vi "Measure S-Param.vi"(4 "error in (no error)":errorcluster, 5 "Array":T1[](array[typedef])=[enum."S11", enum."S12", enum."S21", enum."S22"], 6 "DataFile":path, 7 "Data in":T2 {"LogStartTime" format="%<%x %.3X>T"}) -> (0 "error out":errorcluster, 1 "FileSaved":bool, 3 "Data Out out":T2 {"LogStartTime" format="%<%x %.3X>T"})   [LabVIEW 2023]
uses:
  controls/UI Data.ctl
  <vilib>/NI/Modbus Library/API/Master/Modbus Master.lvclass
  LibreVNA/LibreVNA.lvclass
  LibreVNA/Types/Trace Enum.ctl
  <userlib>/_OpenG.lib/time/time.llb/openg_time.lvlib
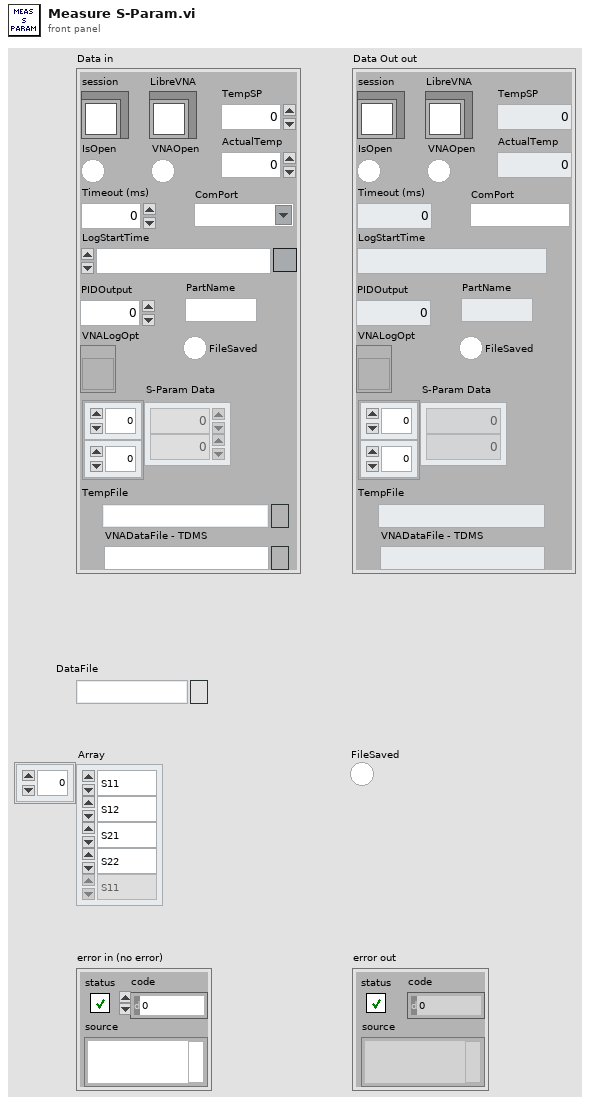
[diagram p1: front panel]
types:
  T1 = typedef "LibreVNA.lvclass/Trace Enum.ctl" = enum16{"S11", "S12", "S21", "S22"}
  T2 = typedef "UI Data.ctl" = cluster{"session":refnum<class "Modbus Master.lvclass">, "IsOpen":bool, "Timeout (ms)":i32, "TempFile":path, "LogStartTime":timestamp, "LibreVNA":refnum<class "LibreVNA.lvclass">, "VNAOpen":bool, "TempSP":dbl, "ActualTemp":dbl, "FileSaved":bool, "PIDOutput":dbl, "VNALogOpt":refnum<vi>, "PartName":string, "ComPort":refnum<visa-resource-name>, "S-Param Data":dbl[][], "VNADataFile - TDMS":path}
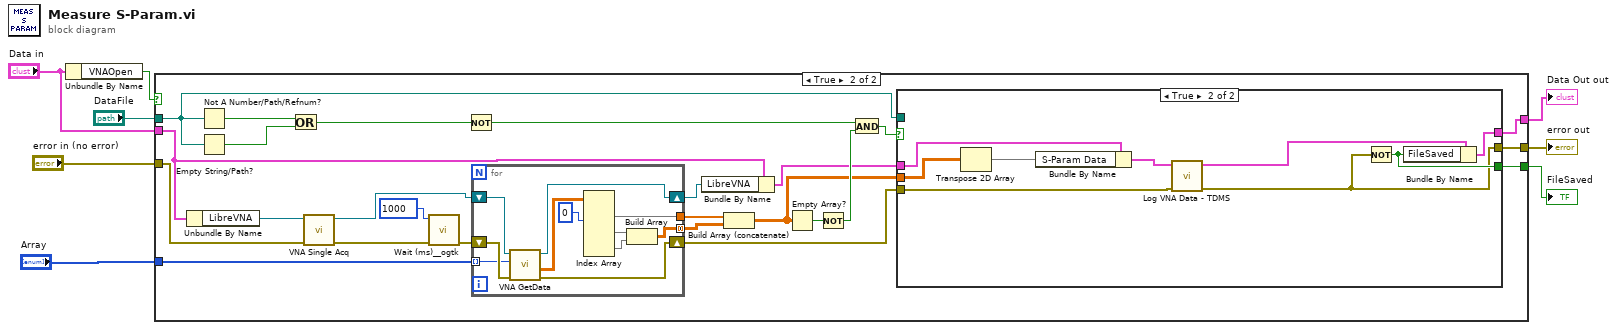
[diagram p0: block diagram]
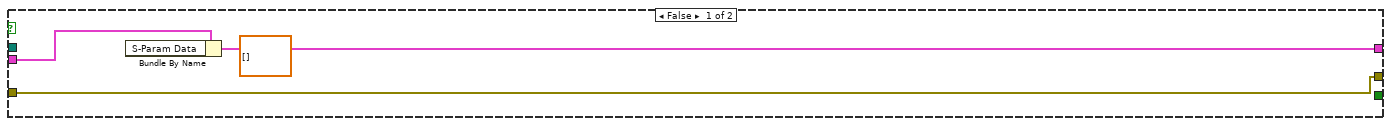
[diagram p2: hidden frame]
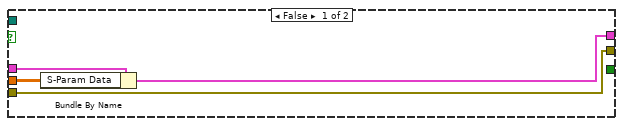
[diagram p3: hidden frame]
diagram:
  n1 = Unbundle By Name("Data in") -> ("VNAOpen"=w6:bool)
  n2 = case shown="True" w6 {
    tunnel: "error in (no error)" -> [w12 w23]
    tunnel: [w12 w25] -> w7
    tunnel: "Array" -> [_ w37]
    tunnel: "DataFile" -> [_ w26]
    tunnel: [_ w24] -> w3
    tunnel: "Data in" -> [w11 w15]
    tunnel: [w10 w18] -> w1
    frame False {
      n3 = Bundle By Name(cluster=w11, "S-Param Data"=dbl[][] []) -> (w10:T2)
    }
    frame True {
      n4 = Unbundle By Name(w15) -> ("LibreVNA"=w14:refnum<class "LibreVNA.lvclass">)
      n5 = Not A Number/Path/Refnum?(number/path/refnum=w26) -> (NaN/Path/Refnum?=w34:bool)
      n6 = Empty String/Path?(string/path=w26) -> (empty?=w33:bool)
      n7 = Or(x=w34, y=w33) -> (x .or. y?=w32:bool)
      n8 = call-dynamic "VNA Single Acq.vi"("error in (no error)"=w23, "LibreVNA in"=w14) -> ("error out"=w21:errorcluster, "LibreVNA out"=w22:refnum<class "LibreVNA.lvclass">)  [unwired: 7 in, 1 out]
      n9 = call <userlib>:"Wait (ms)__ogtk.vi"("error in (no error)"=w21, "milliseconds to wait"=u32 1000) -> ("error out"=w20:errorcluster)  [unwired: 8 in, 1 out]
      n10 = Not(x=w32) -> (.not. x?=w29:bool)
      n11 = for {
        shift-right: [w61] -> w16
        shift-left: w22 -> [w60]
        shift-right: [w58] -> w13
        shift-left: w20 -> [w59]
        tunnel: w37 -> [w57] mode=indexing
        tunnel: [w54] -> w36
        tunnel: [w52] -> w35 mode=concatenating
        n12 = call-dynamic "VNA GetData.vi"("error in (no error)"=w59, "Trace Name"=w57, "LibreVNA in"=w60) -> ("error out"=w58:errorcluster, "Data Out"=w56:dbl[][], "LibreVNA out"=w61:refnum<class "LibreVNA.lvclass">)  [unwired: 3 in, 3 out]
        n13 = Index Array(array=w56, index (col) #1=0 ("disabled index (col)")) -> (element #1=w54:dbl[], element #2=w53:dbl[], element #3=w51:dbl[])  [unwired: 5 in]
        n14 = Build Array(w53, w51) -> (w52:dbl[][])
      }
      n15 = Bundle By Name(cluster=w15, "LibreVNA"=w16) -> (w17:T2)
      n16 = Build Array (concatenate)(w36, w35) -> (w27:dbl[][])
      n17 = Empty Array?(array=w27) -> (empty?=w31:bool)
      n18 = Not(x=w31) -> (.not. x?=w30:bool)
      n19 = And(x=w29, y=w30) -> (x .and. y?=w28:bool)
      n20 = case shown="True" w28 {
        tunnel: w27 -> [w38 w49]
        tunnel: w26 -> [_ _]
        tunnel: w13 -> [w41 w50]
        tunnel: [w41 w43] -> w25
        tunnel: [_ w46] -> w24
        tunnel: w17 -> [w40 w48]
        tunnel: [w39 w47] -> w18
        frame False {
          n21 = Bundle By Name(cluster=w40, "S-Param Data"=w38) -> (w39:T2)
        }
        frame True {
          n22 = Transpose 2D Array(2D array=w49) -> (transposed array=w45:dbl[][])
          n23 = Bundle By Name(cluster=w48, "S-Param Data"=w45) -> (w44:T2)
          n24 = call "Log VNA Data - TDMS.vi"("error in (no error)"=w50, "Data in"=w44) -> ("error out"=w43:errorcluster, "Data out"=w42:T2)  [unwired: 4 in]
          n25 = Not(x=w43) -> (.not. x?=w46:bool)
          n26 = Bundle By Name(cluster=w42, "FileSaved"=w46) -> (w47:T2)
        }
      }
    }
  }
  "Data Out out" <- w1
  "error out" <- w7
  "FileSaved" <- w3
